vi "Read Objects1.vi"(8 "error in (no error)":errorcluster, 11 "device data model in":refnum<class "Standard Data Model1.lvclass">) -> (0 "error out":errorcluster, 2 "objects":cluster{"object ID":u8, "value":string}[](array[cluster]) {"object ID" format="%x"}, 3 "device data model out":refnum<class "Standard Data Model1.lvclass">)   [LabVIEW 2019, in "NI_modbus_upd.lvlib" / "Standard Data Model1.lvclass"]
doc: "Retrieves objects from the device model."
uses:
  Standard Data Model1.lvclass
  Standard Data Model1.lvclass/Standard Data Model1.ctl
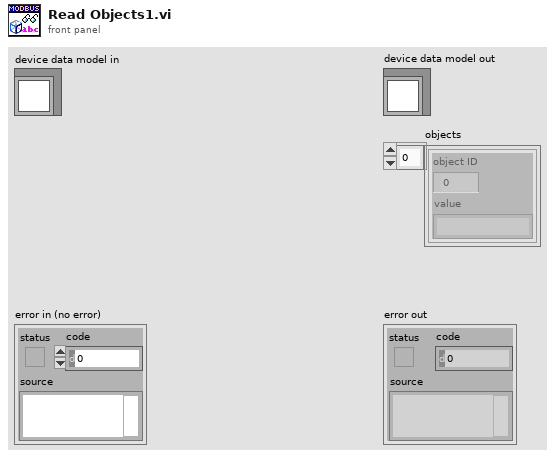
[diagram p1: front panel]
types:
  T1 = typedef "Identification Parameters1.ctl" = cluster{"object ID":u8, "value":string}
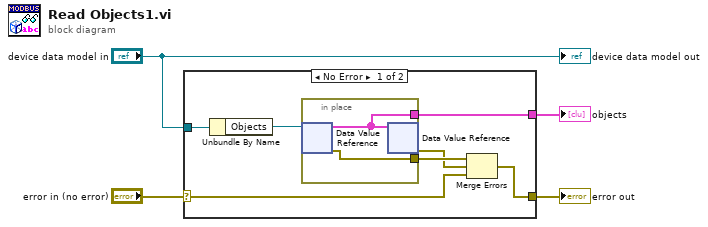
[diagram p0: block diagram]
diagram:
  n1 = case shown="No Error" "error in (no error)" {
    selector: "error in (no error)" -> [w6 w14]
    tunnel: "device data model in" -> [w11 _]
    tunnel: [w9 w14] -> w3
    tunnel: [w8 _] -> w2
    frame No Error {
      n2 = Unbundle By Name(w11) -> ("Objects"=w10:refnum<data-value>)
      n3 = in-place {
        in-place-border: [w13] -> w8
        in-place-border: [w12] -> w7
        n4 = in-place-dvr #1(w10) -> (w13:T1[], w12:errorcluster)
        n5 = in-place-dvr #1(w13) -> (w5:errorcluster)  [unwired: 1 out]
      }
      n6 = Merge Errors(w7, w5, w6) -> (w9:errorcluster)
    }
    frame Error {
    }
  }
  "error out" <- w3
  "objects" <- w2
  "device data model out" <- "device data model in"
